vi "MakeExample.vi"(8 "error in (no error)":errorcluster, 9 "TriggerRefractoryPeriod (Frames)":i32, 10 "StimulusObject Parameters":variant, 11 "HeadandTailRailswithDelay in":refnum<class "HeadandTailRailswithDelay.lvclass">) -> (0 "error out":errorcluster, 3 "HeadandTailRailswithDelay out":refnum<class "HeadandTailRailswithDelay.lvclass">)   [LabVIEW 2019, in "HeadandTailRailswithDelay.lvclass"]
uses:
  HeadandTailRailswithDelay.lvclass
  HeadandTailRailswithDelayInputCluster.ctl
  HeadandTailRailswithDelay.lvclass/HeadandTailRailswithDelay.ctl
  ParametersGlobal.vi
  StimulusObject.lvclass
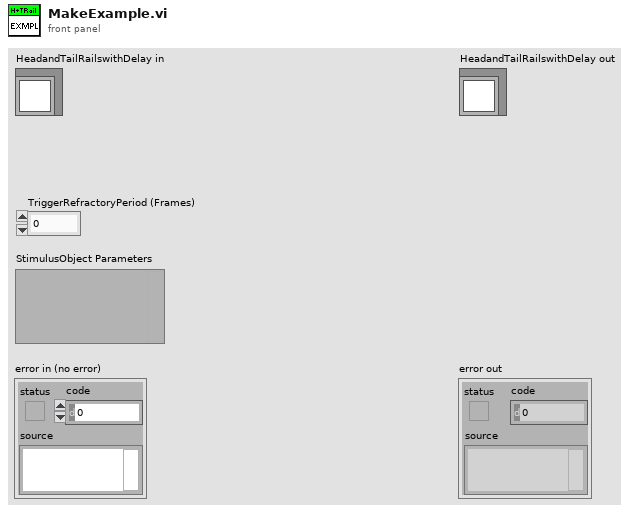
[diagram p1: front panel]
types:
  T1 = typedef "HeadandTailRailswithDelay.lvclass/HeadandTailRailswithDelayInputCluster.ctl" = cluster{"Constant Intensity (uW/mm^2, negative is blue)":sgl, "dot radius (mm)":sgl, "Intensities (uW/mm^2, negative is blue)":sgl[], "Durations (s)":sgl[], "Inter trigger interval (s)":dbl, "Delays (s)":sgl[]}
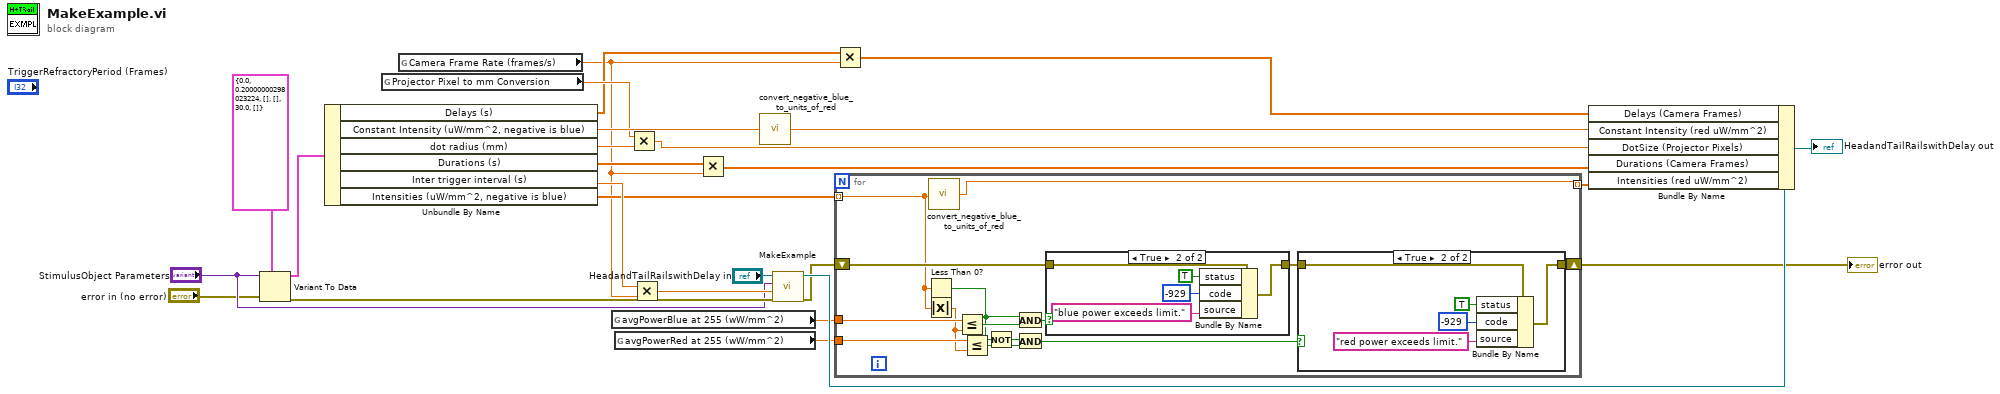
[diagram p0: block diagram]
diagram:
  n1 = Variant To Data(error in="error in (no error)", type=T1 {"Constant Intensity (uW/mm^2, negative is blue)"=0.0, "dot radius (mm)"=0.2, "Intensities (uW/mm^2, negative is blue)"=[], "Durations (s)"=[], "Inter trigger interval (s)"=30.0, "Delays (s)"=[]} ("JustHeadsRailsInputCluster"), Variant="StimulusObject Parameters") -> (data=w25:T1, error out=w26:errorcluster)
  n2 = Unbundle By Name(w25) -> ("Delays (s)"=w3:sgl[], "Constant Intensity (uW/mm^2, negative is blue)"=w21:sgl, "dot radius (mm)"=w19:sgl, "Durations (s)"=w16:sgl[], "Inter trigger interval (s)"=w24:dbl, "Intensities (uW/mm^2, negative is blue)"=w14:sgl[])
  n3 = global read "ParametersGlobal.vi" "Projector Pixel to mm Conversion"() -> (w18:sgl)
  n4 = global read "ParametersGlobal.vi" "Camera Frame Rate (frames/s)"() -> (w2:sgl)
  n5 = global read "ParametersGlobal.vi" "avgPowerBlue at 255 (wW/mm^2)"() -> (w12:sgl)
  n6 = global read "ParametersGlobal.vi" "avgPowerRed at 255 (wW/mm^2)"() -> (w11:sgl)
  n7 = Multiply(x=w18, y=w19) -> (x*y=w17:sgl)
  n8 = Multiply(x=w24, y=w2) -> (x*y=w23:dbl)
  n9 = Multiply(x=w16, y=w2) -> (x*y=w15:sgl[])
  n10 = call "convert_negative_blue_to_units_of_red.vi"("Intensity in units of red (positive) and blue (negative)"=w21) -> ("Intensity in units of red (positive and negative)"=w20:sgl)
  n11 = call-parent "MakeExample.vi"("error in (no error)"=w26, "TriggerRefractoryPeriod (Frames)"=w23, "StimulusObject Parameters"="StimulusObject Parameters", "StimulusObject in"="HeadandTailRailswithDelay in") -> ("error out"=w13:errorcluster, "StimulusObject out"=w22:refnum<class "HeadandTailRailswithDelay.lvclass">)  [unwired: 6 in]
  n12 = Multiply(x=w3, y=w2) -> (x*y=w1:sgl[])
  n13 = for {
    tunnel: w14 -> [w34] mode=indexing
    shift-right: [w38] -> w5
    shift-left: w13 -> [w39]
    tunnel: w12 -> [w37]
    tunnel: w11 -> [w36]
    tunnel: [w35] -> w10 mode=indexing
    n14 = Less Than 0?(x=w34) -> (x < 0?=w27:bool)
    n15 = Absolute Value(x=w34) -> (abs(x)=w33:sgl)
    n16 = call "convert_negative_blue_to_units_of_red.vi"("Intensity in units of red (positive) and blue (negative)"=w34) -> ("Intensity in units of red (positive and negative)"=w35:sgl)
    n17 = Less Or Equal?(x=w37, y=w33) -> (x <= y?=w32:bool)
    n18 = Less Or Equal?(x=w36, y=w33) -> (x <= y?=w29:bool)
    n19 = Not(x=w27) -> (.not. x?=w28:bool)
    n20 = And(x=w27, y=w32) -> (x .and. y?=w31:bool)
    n21 = And(x=w28, y=w29) -> (x .and. y?=w30:bool)
    n22 = case shown="True" w31 {
      tunnel: w39 -> [w47 w52]
      tunnel: [w47 w51] -> w40
      frame False {
      }
      frame True {
        n23 = Bundle By Name(cluster=w52, "status"=TRUE, "code"=-929, "source"="blue power exceeds limit.") -> (w51:errorcluster)
      }
    }
    n24 = case shown="True" w30 {
      tunnel: w40 -> [w41 w46]
      tunnel: [w41 w45] -> w38
      frame False {
      }
      frame True {
        n25 = Bundle By Name(cluster=w46, "status"=TRUE, "code"=-929, "source"="red power exceeds limit.") -> (w45:errorcluster)
      }
    }
  }
  "error out" <- w5
  n26 = Bundle By Name(cluster=w22, "Delays (Camera Frames)"=w1, "Constant Intensity (red uW/mm^2)"=w20, "DotSize (Projector Pixels)"=w17, "Durations (Camera Frames)"=w15, "Intensities (red uW/mm^2)"=w10) -> (→"HeadandTailRailswithDelay out":refnum<class "HeadandTailRailswithDelay.lvclass">)
